vi "Relu.vi"(10 "Data In":dbl[](array[numeric])) -> (2 "Data out":dbl[](array[numeric]))   [LabVIEW 2018]
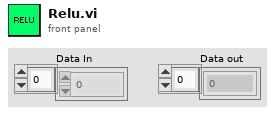
[diagram p1: front panel]
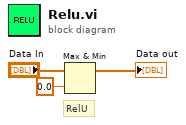
[diagram p0: block diagram]
diagram:
  # "RelU"
  n1 = Max & Min(x="Data In", y=0.0) -> (max(x,y)=→"Data out":dbl[])  [unwired: 1 out]
